vi "Exercises_5-1-1.vi"() -> ()   [LabVIEW 2014]
panel:
  out "Intensity Graph":dbl[][](graph)
  out "Array":dbl[][](array[numeric])
  in  "Colums":i32
  in  "Rows":i32
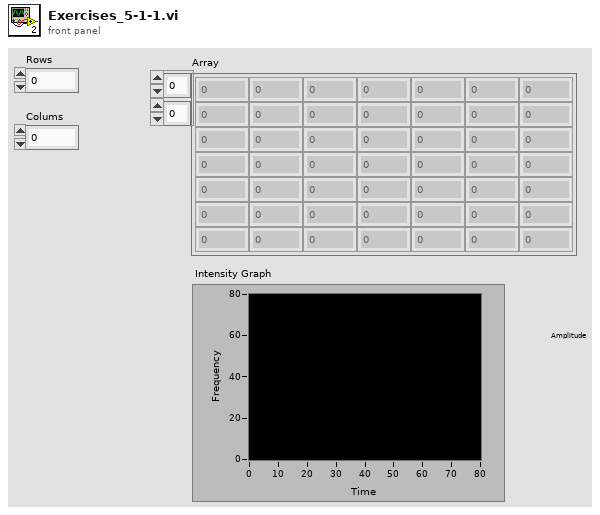
[diagram p1: front panel]
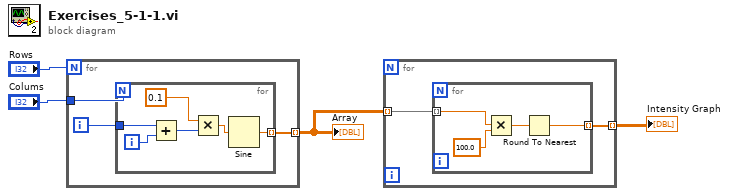
[diagram p0: block diagram]
diagram:
  n1 = for {
    N: "Rows" -> [_]
    tunnel: "Colums" -> [w7]
    tunnel: [w5] -> w2 mode=indexing
    i -> [w6]
    n2 = for {
      N: w7 -> [_]
      tunnel: w6 -> [w13]
      tunnel: [w8] -> w5 mode=indexing
      i -> [w12]
      n3 = Add(x=w13, y=w12) -> (x+y=w10:i32)
      n4 = Multiply(x=0.1, y=w10) -> (x*y=w9:dbl)
      n5 = Sine(x=w9) -> (sin(x)=w8:dbl)
    }
  }
  "Array" <- w2
  n6 = for {
    tunnel: w2 -> [w15] mode=indexing
    tunnel: [w14] -> w1 mode=indexing
    n7 = for {
      tunnel: w15 -> [w18] mode=indexing
      tunnel: [w16] -> w14 mode=indexing
      n8 = Multiply(x=w18, y=100.0) -> (x*y=w17:dbl)
      n9 = Round To Nearest(number=w17) -> (nearest integer value=w16:dbl)
    }
  }
  "Intensity Graph" <- w1
